vi "Read Result.vi"(8 "error in (no error)":errorcluster, 11 "SimpleArithmetic in":refnum<class "SimpleArithmetic.lvclass">) -> (0 "error out":errorcluster, 2 "Result":dbl, 3 "SimpleArithmetic out":refnum<class "SimpleArithmetic.lvclass">)   [LabVIEW 2011, in "SimpleArithmetic.lvclass"]
uses:
  SimpleArithmetic.lvclass
  SimpleArithmetic.lvclass/SimpleArithmetic.ctl
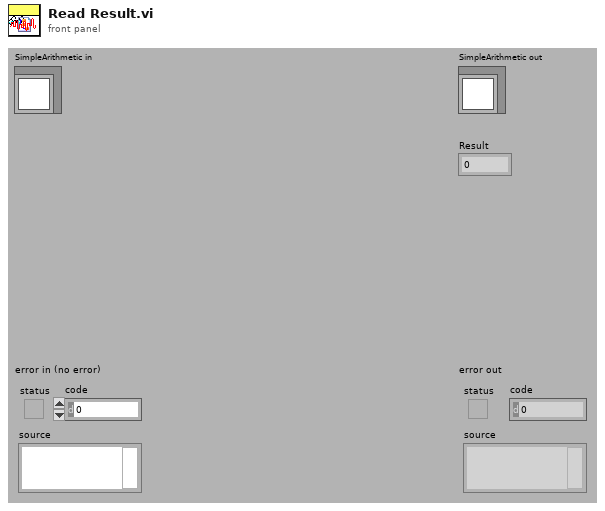
[diagram p1: front panel]
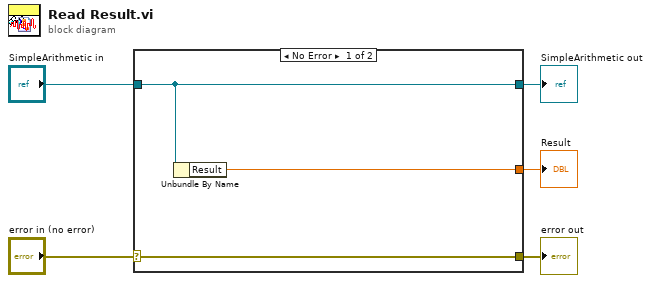
[diagram p0: block diagram]
diagram:
  n1 = case shown="No Error" "error in (no error)" {
    selector: "error in (no error)" -> [w8 w9]
    tunnel: [w8 w9] -> w4
    tunnel: [w7 w10] -> w2
    tunnel: "SimpleArithmetic in" -> [w7 w10]
    tunnel: [w6 _] -> w1
    frame No Error {
      n2 = Unbundle By Name(w7) -> ("Result"=w6:dbl)
    }
    frame Error {
    }
  }
  "error out" <- w4
  "SimpleArithmetic out" <- w2
  "Result" <- w1
